vi "EditValue.vi"(8 "error in (no error)":errorcluster, 10 "Bounds":T1, 11 "U32 D Element.lvclass":refnum<class "U8 D Element.lvclass">) -> (0 "error out":errorcluster, 1 "Tabbed out?":bool, 2 "Value changed?":bool, 3 "U32 D Element.lvclass":refnum<class "U8 D Element.lvclass">)   [LabVIEW 2018, in "D Datagrid Library.lvlib" / "U8 D Element.lvclass"]
uses:
  U8 D Element.lvclass
  <vilib>/Utility/miscctls.llb/LVRectTypeDef.ctl
  U8 D Element.lvclass/U8 D Element.ctl
  Read Display mode.vi
panel:
  in  "Value":u8 format="%.0x"
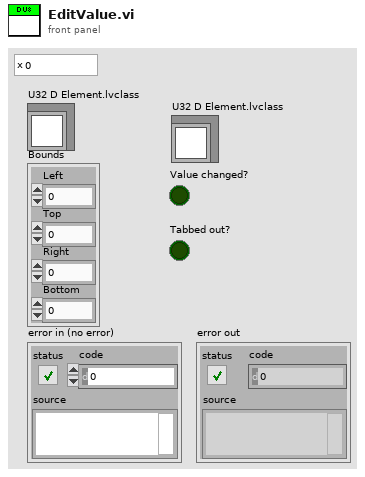
[diagram p1: front panel]
types:
  T1 = typedef "LVRectTypeDef.ctl" = cluster{"Left":i16, "Top":i16, "Right":i16, "Bottom":i16}
  T2 = typedef "D Datagrid Library.lvlib/U32 D Element.lvclass/Display mode.ctl" = enum16{"Standard", "Hex"}
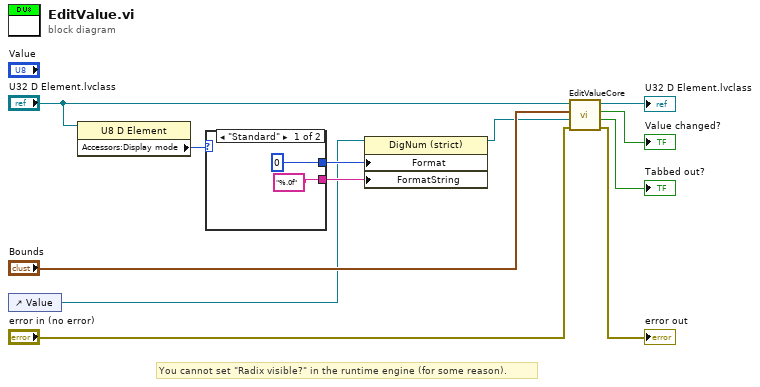
[diagram p0: block diagram]
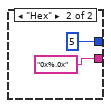
[diagram p2: hidden frame]
diagram:
  # "You cannot set \"Radix visible?\" in the runtime engine (for some reason)."
  n1 = control-ref of="Value"() -> (w3:refnum<vi>)
  n2 = property class="U8 D Element"(reference="U32 D Element.lvclass") -> ("Accessors:Display mode"=w4:T2)  [unwired: 1 in, 2 out]
  n3 = case shown="\"Standard\"" w4 {
    tunnel: [u8 0 ("Display Format:Format") u8 5 ("Display Format:Format")] -> w6
    tunnel: ["%.0f" "0x%.0x"] -> w5
    frame "Standard" {
    }
    frame "Hex" {
    }
  }
  n4 = property class="DigNum (strict)"(reference=w3, "Format"=w6, "FormatString"=w5) -> (reference out=w2:refnum<vi>)  [unwired: 1 in, 1 out]
  n5 = call-dynamic "EditValueCore.vi"("error in (no error)"="error in (no error)", "Value field reference"=w2, "Bounds"="Bounds", "DatagridElement in"="U32 D Element.lvclass") -> ("error out"=→"error out":errorcluster, "Tabbed out?"=→"Tabbed out?":bool, "Value changed?"=→"Value changed?":bool, "DatagridElement out"=→"U32 D Element.lvclass":refnum<class "U8 D Element.lvclass">)  [unwired: 4 in]
